vi "split_bin_string.vi"(11 "String":string) -> (1 "Fraction":u8[](array[numeric]), 2 "Integer":u8[](array[numeric]), 3 "Sign":u8)   [LabVIEW 2025]
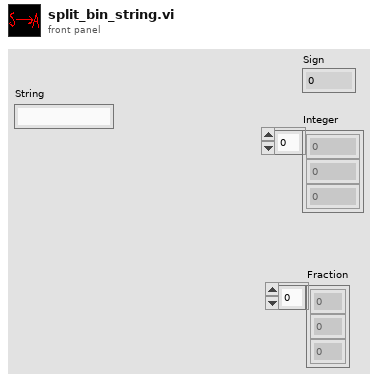
[diagram p1: front panel]
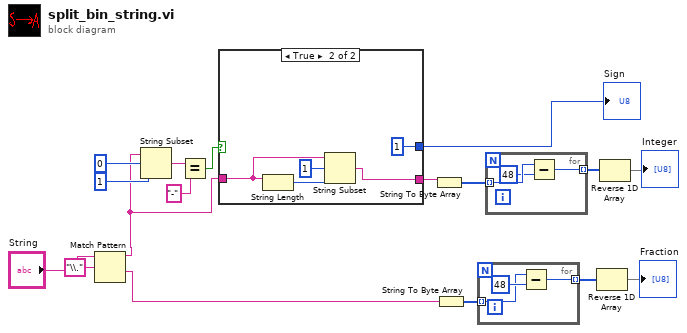
[diagram p0: block diagram]
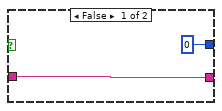
[diagram p2: hidden frame]
diagram:
  n1 = Match Pattern(string="String", regular expression="\\.") -> (before substring=w8:string, after substring=w7:string)  [unwired: 1 in, 2 out]
  n2 = String Subset(string=w8, offset (0)=0, length (rest)=1 ("length (rest)")) -> (substring=w13:string)
  n3 = Equal?(x=w13, y="-") -> (x = y?=w11:bool)
  n4 = case shown="True" w11 {
    tunnel: [u8 0 u8 1] -> w10
    tunnel: w8 -> [w18 w22]
    tunnel: [w18 w20] -> w9
    frame False {
    }
    frame True {
      n5 = String Length(string=w22) -> (length=w21:i32)
      n6 = String Subset(string=w22, offset (0)=1, length (rest)=w21) -> (substring=w20:string)
    }
  }
  "Sign" <- w10
  n7 = String To Byte Array(string=w9) -> (unsigned byte array=w6:u8[])
  n8 = String To Byte Array(string=w7) -> (unsigned byte array=w5:u8[])
  n9 = for {
    tunnel: [w26] -> w2 mode=indexing
    tunnel: w5 -> [w25] mode=indexing
    n10 = Subtract(x=w25, y=u8 48) -> (x-y=w26:u8)
  }
  n11 = for {
    tunnel: w6 -> [w30] mode=indexing
    tunnel: [w28] -> w4 mode=indexing
    n12 = Subtract(x=w30, y=u8 48) -> (x-y=w28:u8)
  }
  n13 = Reverse 1D Array(array=w2) -> (reversed array=→"Fraction":u8[])
  n14 = Reverse 1D Array(array=w4) -> (reversed array=→"Integer":u8[])
